vi "FT10_M4X Status.vi"(11 "Card Handle in":u32) -> (2 "Ready?":bool, 3 "Card Handle out":u32)   [LabVIEW 2015]
doc: "Copy of \"M4X_Status.vi\" from HWT_Lillis_7854.lvproj"
uses:
  spcm_win32.dll
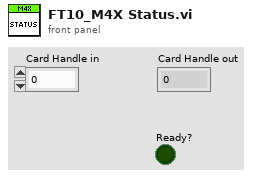
[diagram p1: front panel]
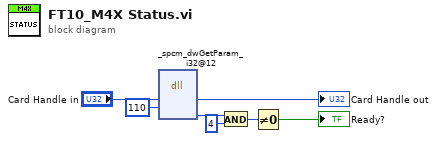
[diagram p0: block diagram]
diagram:
  n1 = dll-call lib="spcm_win32.dll" fn="_spcm_dwGetParam_i32@12"("hDrv"="Card Handle in", "lRegister"=110) -> ("hDrv"=→"Card Handle out":u32, "lValue"=w4:i32)  [unwired: 6 in, 2 out]
  n2 = And(x=w4, y=4) -> (x .and. y?=w6:i32)
  n3 = Not Equal To 0?(x=w6) -> (x != 0?=→"Ready?":bool)
